vi "table重新排序.vi"(11 "tables":string[](array[string])) -> (3 "sorted elements":string[](array[string]))   [LabVIEW 2016, in "数据查询.lvlib"]
uses:
  <userlib>/_OpenG.lib/array/array.llb/Delete Elements from 1D Array (String)__ogtk.vi
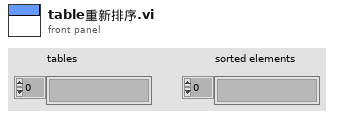
[diagram p1: front panel]
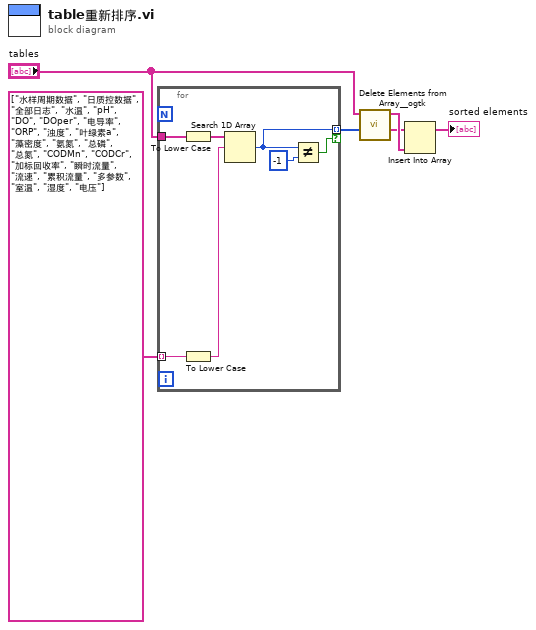
[diagram p0: block diagram]
diagram:
  n1 = for {
    tunnel: "tables" -> [w11]
    tunnel: string[] ["水样周期数据", "日质控数据", "全部日志", "水温", "pH", "DO", "DOper", "电导率", "ORP", "浊度", "叶绿素a", "藻密度", "氨氮", "总磷", "总氮", "CODMn", "CODCr", "加标回收率", "瞬时流量", "流速", "累积流量", "多参数", "室温", "湿度", "电压"] ("tables") -> [w13] mode=indexing
    tunnel: [w10] -> w4 mode=indexing if=w9
    n2 = To Lower Case(string=w11) -> (all lower case string=w8:string[])
    n3 = To Lower Case(string=w13) -> (all lower case string=w7:string)
    n4 = Search 1D Array(1D array=w8, element=w7) -> (index of element=w10:i32)  [unwired: 1 in]
    n5 = Not Equal?(x=w10, y=-1) -> (x != y?=w9:bool)
  }
  n6 = call-poly <userlib>:"Delete Elements from Array__ogtk.vi"("indices"=w4, "array"="tables") -> ("deleted elements"=w5:string[], "array w/ subset deleted"=w6:string[])  [unwired: 8 in]
  n7 = Insert Into Array(array=w5, new element=w6) -> (→"sorted elements":string[])  [unwired: 1 in]
